vi "updateSWupdateLog.vi"(7 "name or relative path":string="EnFloSWupdateLog.txt", 10 "currentRevisions":string[](array[string]), 11 "log file path (local default if blank)":path) -> ()   [LabVIEW 2021]
uses:
  <vilib>/Utility/file.llb/Write Delimited Spreadsheet (string).vi
  <vilib>/Utility/file.llb/Read Delimited Spreadsheet (string).vi
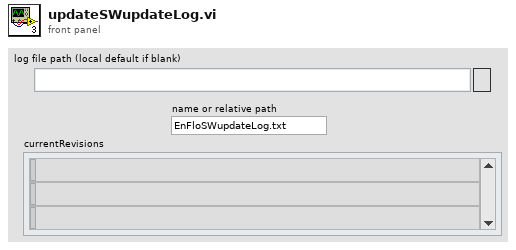
[diagram p1: front panel]
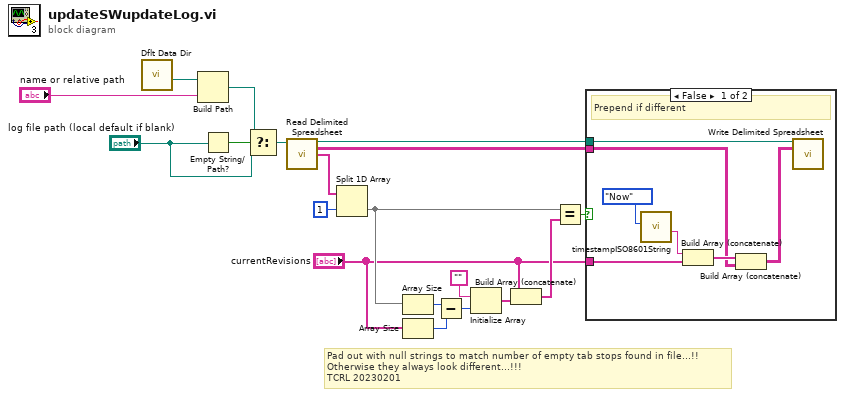
[diagram p0: block diagram]
diagram:
  # "Pad out with null strings to match number of empty tab stops found in file...!!\nOtherwise they always look different...!!!\nTCRL 20230201"
  n1 = call <vilib>:"Dflt Data Dir.vi"() -> ("App:Default Data Directory"=w18:path)
  n2 = Build Path(base path=w18, name or relative path="name or relative path") -> (appended path=w15:path)
  n3 = Empty String/Path?(string/path="log file path (local default if blank)") -> (empty?=w17:bool)
  n4 = Select(t=w15, s=w17, f="log file path (local default if blank)") -> (s? t:f=w11:path)
  n5 = call-poly <vilib>:"Read Delimited Spreadsheet.vi"("file path (dialog if empty)"=w11) -> ("new file path (Not A Path if cancelled)"=w10:path, "all rows"=w12:string[][], "first row"=w14:string[])  [unwired: 9 in, 3 out]
  n6 = Split 1D Array(array=w14, index=1) -> (second subarray=w9:string[])  [unwired: 1 out]
  n7 = Array Size(array=w9) -> (size(s)=w6:i32)
  n8 = Array Size(array="currentRevisions") -> (size(s)=w5:i32)
  n9 = Subtract(x=w6, y=w5) -> (x-y=w4:i32)
  n10 = Initialize Array("", w4) -> (w3:string[])
  n11 = Build Array (concatenate)("currentRevisions", w3) -> (w2:string[])
  n12 = Equal?(x=w9, y=w2) -> (x = y?=w7:bool)
  n13 = case shown="False" w7 {
    tunnel: w12 -> [w22 _]
    tunnel: "currentRevisions" -> [w26 _]
    tunnel: w10 -> [w24 _]
    frame False {
      # "Prepend if different"
      n14 = call "timestampISO8601String.vi"("When?"=enum16{"Now", "Use Input"}."Now") -> ("date/time"=w25:string)  [unwired: 7 in, 3 out]
      n15 = Build Array (concatenate)(w25, w26) -> (w23:string[])
      n16 = Build Array (concatenate)(w23, w22) -> (w21:string[][])
      n17 = call-poly <vilib>:"Write Delimited Spreadsheet.vi"("file path (dialog if empty)"=w24, "2D data"=w21) -> ()  [unwired: 12 in, 2 out]
    }
    frame True {
    }
  }
